vi "Write Transient Sheet.vi"(8 "error in (no error)":errorcluster, 10 "Data Analyser Report.lvclass":refnum<class "Data Analyser Report.lvclass">, 11 "Excel Logger in":refnum<class "Excel Logger.lvclass">) -> (0 "error out":errorcluster, 3 "Excel Logger out":refnum<class "Excel Logger.lvclass">)   [LabVIEW 2013, in "Excel Logger.lvclass"]
uses:
  Excel Logger.lvclass
  Data Analyser Report/Data Analyser Report.lvclass
  Excel Logger.lvclass/Excel Logger.ctl
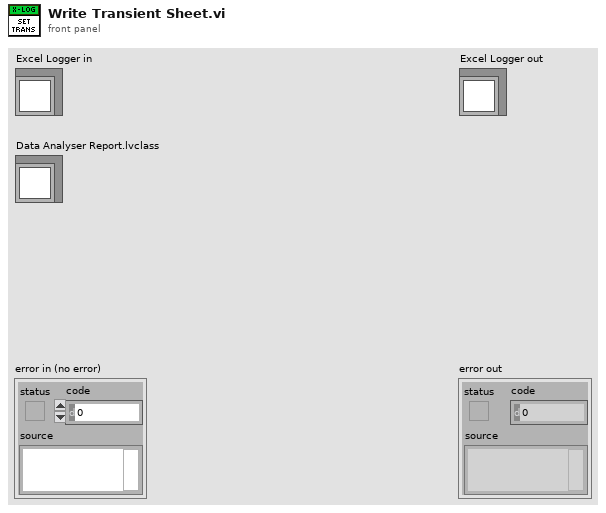
[diagram p1: front panel]
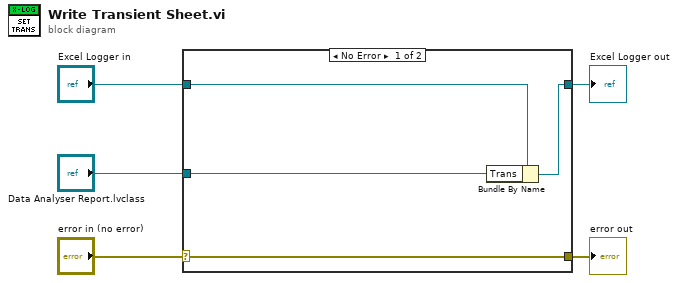
[diagram p0: block diagram]
diagram:
  n1 = case shown="No Error" "error in (no error)" {
    selector: "error in (no error)" -> [w9 w10]
    tunnel: [w9 w10] -> w4
    tunnel: [w7 w11] -> w2
    tunnel: "Excel Logger in" -> [w8 w11]
    tunnel: "Data Analyser Report.lvclass" -> [w6 _]
    frame No Error {
      n2 = Bundle By Name(cluster=w8, "Trans"=w6) -> (w7:refnum<class "Excel Logger.lvclass">)
    }
    frame Error {
    }
  }
  "error out" <- w4
  "Excel Logger out" <- w2
